vi "Tophat Init LUT.vi"(7 "Number of  Elements":i32=80000, 8 "Df":i16=200, 9 "f0":i16=1350) -> (3 "Init Data Out":i16[](array[numeric]))   [LabVIEW 2018]
uses:
  <vilib>/Analysis/2dsp.llb/Inverse Real FFT.vi
  <vilib>/Analysis/NI_AALPro.lvlib
panel:
  out "f(t) half":i32[](graph)
  out "min value":i32=-32360
  out "max value":i32=-32768
  out "f(t)":i32[](graph)
  out "Frequency Domain Signal":i64[](graph)
  # "This is the max number of elements that will sit in a 16 bit wide block of memory"
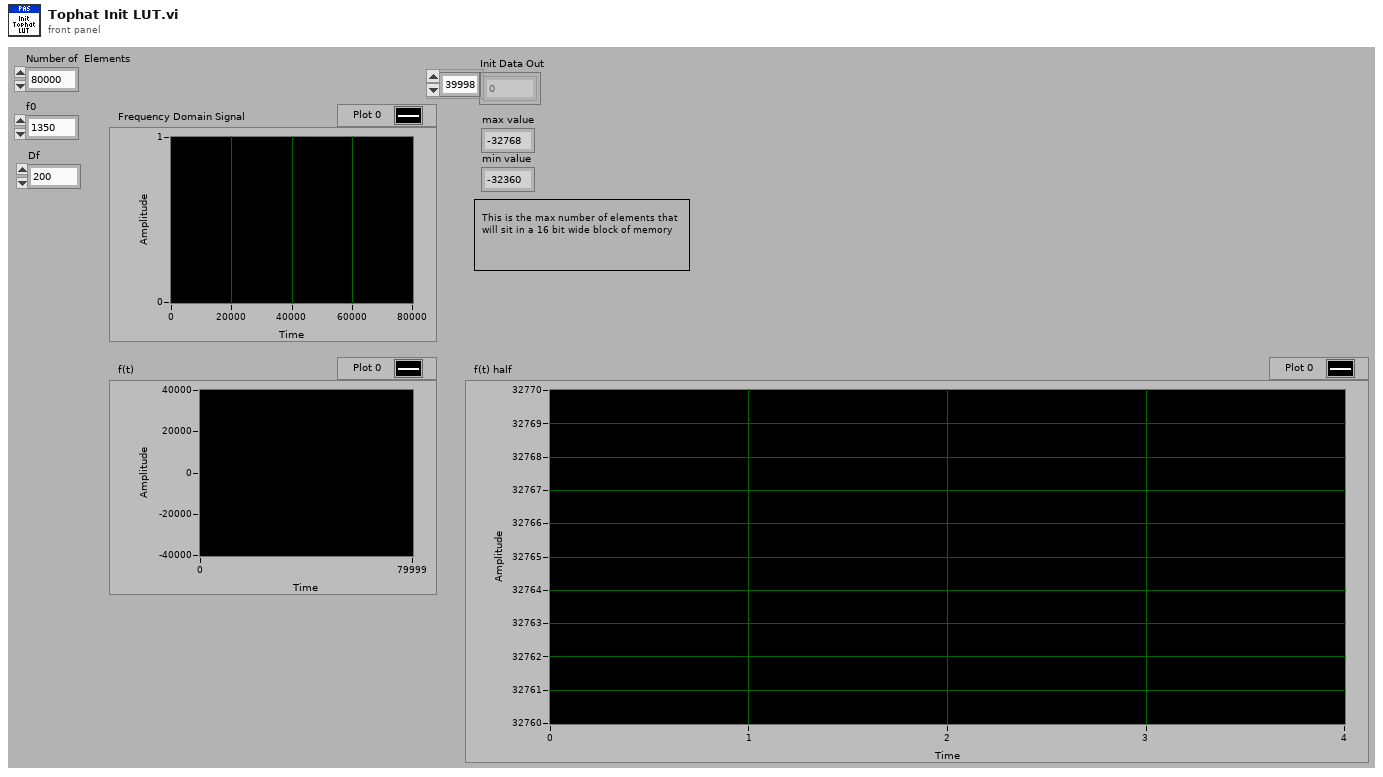
[diagram p1: front panel]
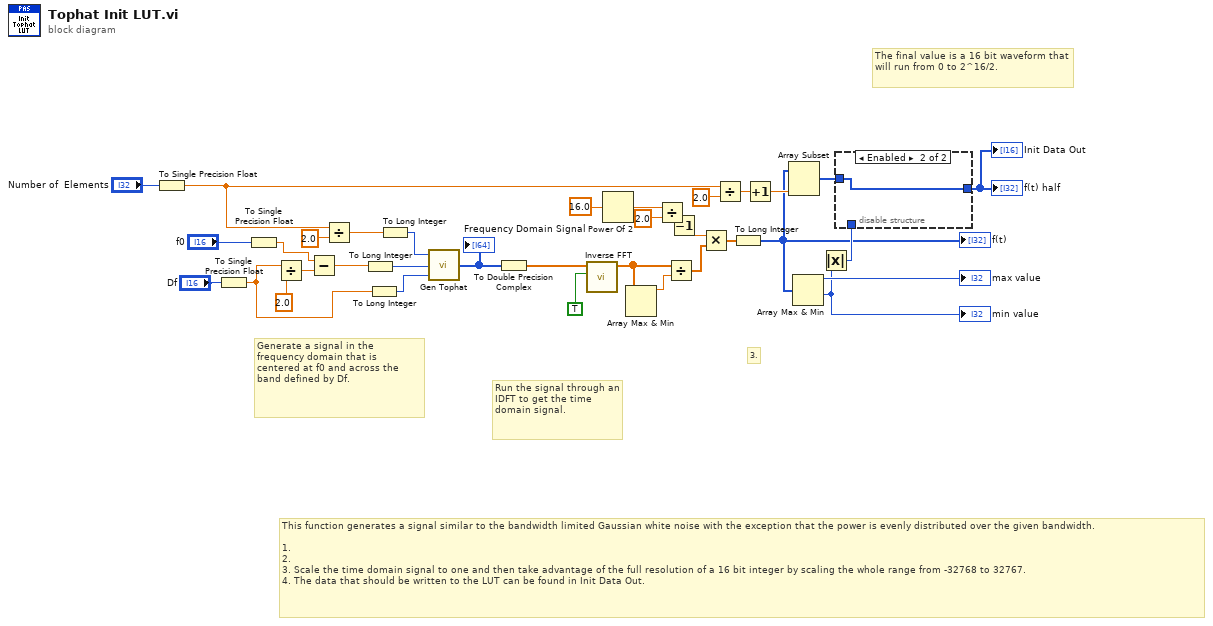
[diagram p0: block diagram]
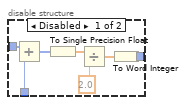
[diagram p2: hidden frame]
diagram:
  # "The final value is a 16 bit waveform that will run from 0 to 2^16/2."
  # "Generate a signal in the frequency domain that is centered at f0 and across the band defined by Df."
  # "3."
  # "Run the signal through an IDFT to get the time domain signal."
  # "This function generates a signal similar to the bandwidth limited Gaussian white noise with the exception that the power is evenly distributed over the given bandwidth.\n\n1. \n2. \n3. Scale the time domain signal to one and then take advantage of the full resolution of a 16 bit integer by scaling the whole range from -32768 to 32767.\n4. The data that should be written to the LUT can be found in Init Data Out."
  n1 = To Single Precision Float(number="Number of  Elements") -> (single precision float=w10:sgl)
  n2 = To Single Precision Float(number="Df") -> (single precision float=w5:sgl)
  n3 = To Single Precision Float(number="f0") -> (single precision float=w12:sgl)
  n4 = Divide(x=w5, y=sgl 2.0) -> (x/y=w27:sgl)
  n5 = Subtract(x=w12, y=w27) -> (x-y=w7:sgl)
  n6 = Divide(x=w10, y=sgl 2.0) -> (x/y=w9:sgl)
  n7 = To Long Integer(number=w7) -> (32bit integer=w6:i32)
  n8 = To Long Integer(number=w5) -> (32bit integer=w4:i32)
  n9 = To Long Integer(number=w9) -> (32bit integer=w8:i32)
  n10 = call "Gen Tophat.vi"("Frequency Span"=w4, "Lower Frequency \nLocation"=w6, "Nyquist Frequency\nLocation"=w8) -> ("Waveform Graph"=w3:i64[])
  "Frequency Domain Signal" <- w3
  n11 = To Double Precision Complex(1:w3) -> (0:w2:cdb[])
  n12 = call-poly <vilib>:"Inverse FFT.vi"("shift?"=TRUE, "FFT {X}"=w2) -> ("X"=w31:dbl[])  [unwired: 9 out]
  n13 = Power Of 2(x=sgl 16.0) -> (2^x=w30:sgl)
  n14 = Array Max & Min(array=w31) -> (max value=w21:dbl)  [unwired: 3 out]
  n15 = Divide(x=w30, y=sgl 2.0) -> (x/y=w28:sgl)
  n16 = Divide(x=w31, y=w21) -> (x/y=w22:dbl[])
  n17 = Decrement(x=w28) -> (x-1=w1:sgl)
  n18 = Multiply(x=w1, y=w22) -> (x*y=w16:dbl[])
  n19 = Divide(x=w10, y=sgl 2.0) -> (x/y=w24:sgl)
  n20 = To Long Integer(number=w16) -> (32bit integer=w15:i32[])
  "f(t)" <- w15
  n21 = Increment(x=w24) -> (x+1=w23:sgl)
  n22 = Array Subset(array=w15, length=w23) -> (w20:i32[])  [unwired: 1 in]
  n23 = Array Max & Min(array=w15) -> (max value=→"max value":i32, min value=w18:i32)  [unwired: 2 out]
  "min value" <- w18
  n24 = Absolute Value(x=w18) -> (abs(x)=w17:i32)
  n25 = disable-structure shown="Enabled" {
    disable-tunnel: w20 -> [w42 w43]
    disable-tunnel: [w39 w43] -> w19
    disable-tunnel: w17 -> [w38 _]
    frame Disabled {
      n26 = Add(x=w42, y=w38) -> (x+y=w37:i32[])
      n27 = To Single Precision Float(number=w37) -> (single precision float=w36:sgl[])
      n28 = Divide(x=w36, y=sgl 2.0) -> (x/y=w40:sgl[])
      n29 = To Word Integer(number=w40) -> (16bit integer=w39:i16[])
    }
    frame Enabled {
    }
  }
  "Init Data Out" <- w19
  "f(t) half" <- w19
